vi "Trigger Source Setting.vi"(8 "error in (no error)":errorcluster, 11 "VISA resource name":refnum<visa-resource-name>) -> (0 "value out":errorcluster, 3 "VISA resource name out":refnum<visa-resource-name>)   [LabVIEW 2025, in "Rigol.lvlib"]
uses:
  Rigol.lvlib
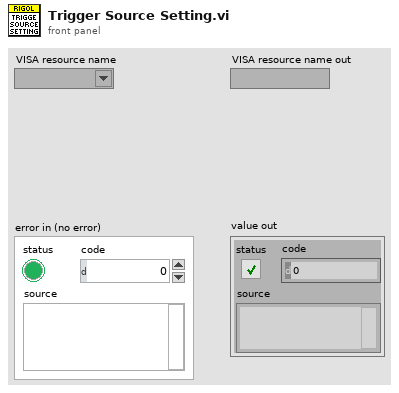
[diagram p1: front panel]
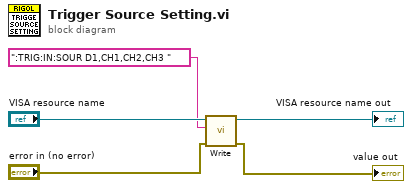
[diagram p0: block diagram]
diagram:
  n1 = call "Write.vi"("error in (no error)"="error in (no error)", "Write Buffer (\"\")"=":TRIG:IN:SOUR D1,CH1,CH2,CH3 " ("format string"), "VISA resource name"="VISA resource name") -> ("error out"=→"value out":errorcluster, "VISA resource name out"=→"VISA resource name out":refnum<visa-resource-name>)  [unwired: 7 in]
